vi "Update Results.vi"(0 "MeasurementServiceV2 in":refnum<class "MeasurementServiceV2.lvclass">, 5 "Measurement Results":variant, 7 "MeasurementPluginService in":refnum<class "MeasurementPluginService.lvclass">, 9 "gRPCid in":T1, 11 "error in (no error)":errorcluster) -> (4 "MeasurementServiceV2 out":refnum<class "MeasurementServiceV2.lvclass">, 8 "MeasurementPluginService out":refnum<class "MeasurementPluginService.lvclass">, 15 "error out":errorcluster)   [LabVIEW 2020, in "MeasurementLink Measurement Server.lvlib" / "MeasurementServiceV2.lvclass"]
uses:
  MeasurementServiceV2.lvclass
  <vilib>/gRPC/LabVIEW gRPC Library/Shared/grpcId.ctl
  MeasurementPluginService/MeasurementPluginService.lvclass
  MeasurementLink Measurement Service Base V2/RPC Messages/ni_measurementlink_measurement_v2_MeasureResponse.ctl
  MeasurementLink Measurement Service Base V2/RPC Messages/google_protobuf_Any.ctl
  MeasurementLink Measurement Service Base V2/RPC Service/MeasurementService/MeasurementServiceBaseV2.lvclass
  MeasurementLink Measurement Service Base V2/MeasurementLink Measurement Service Base V2.lvlib
  <vilib>/gRPC/LabVIEW gRPC Library/grpc-lvsupport-release.lvlib
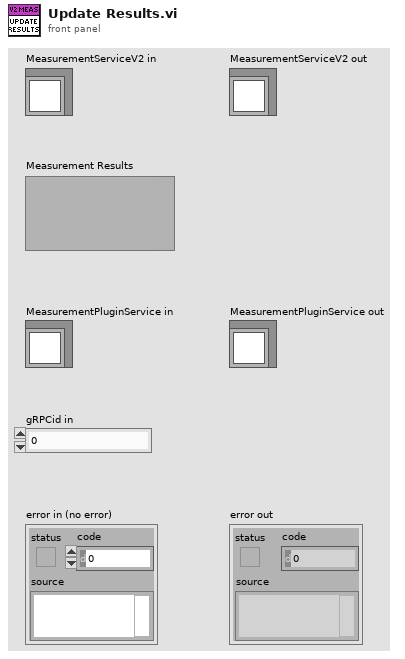
[diagram p1: front panel]
types:
  T1 = typedef "grpc-lvsupport-release.lvlib/grpcId.ctl" = u64
  T2 = typedef "MeasurementLink Measurement Service Base V2.lvlib/ni_measurementlink_measurement_v2_MeasureResponse.ctl" = cluster{"outputs":T3}
  T3 = typedef "MeasurementLink Measurement Service Base V2.lvlib/google_protobuf_Any.ctl" = cluster{"type_url":string, "value":u8[]}
  T4 = typedef "grpc-lvsupport-release.lvlib/Any.ctl" = cluster{"Type Url":string, "Bytes":u8[]}
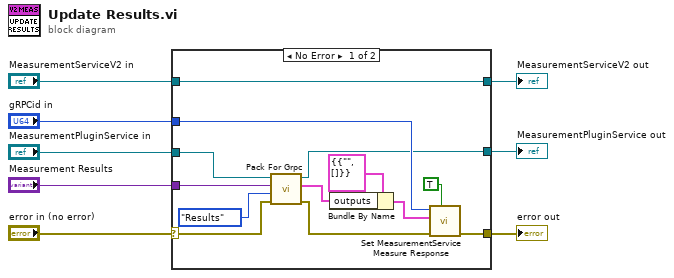
[diagram p0: block diagram]
diagram:
  n1 = case shown="No Error" "error in (no error)" {
    selector: "error in (no error)" -> [w14 w24]
    tunnel: [w21 w24] -> w7
    tunnel: [w18 w23] -> w5
    tunnel: "MeasurementServiceV2 in" -> [w18 w23]
    tunnel: "Measurement Results" -> [w16 _]
    tunnel: "gRPCid in" -> [w19 _]
    tunnel: "MeasurementPluginService in" -> [w17 w22]
    tunnel: [w12 w22] -> w1
    frame No Error {
      n2 = call-dynamic "Pack For Grpc.vi"("error in (no error)"=w14, "Configuration / Resuls (Config)"=enum16{"Configuration", "Results"}."Results", "Data Value"=w16, "MeasurementPluginService in"=w17) -> ("error out"=w13:errorcluster, "Any"=w10:T4, "MeasurementPluginService out"=w12:refnum<class "MeasurementPluginService.lvclass">)  [unwired: 5 in]
      n3 = Bundle By Name(cluster=T2 {"outputs"={"type_url"="", "value"=[]}} ("Message Data"), "outputs"=w10) -> (w9:T2)
      n4 = call "Set MeasurementService Measure Response.vi"("Streaming? (F)"=TRUE, "error in (no error)"=w13, "Message Data"=w9, "gRPCid in"=w19) -> ("error out"=w21:errorcluster)  [unwired: 7 in]
    }
    frame Error {
    }
  }
  "error out" <- w7
  "MeasurementServiceV2 out" <- w5
  "MeasurementPluginService out" <- w1
